vi "Recieve Idot Result.vi"(8 "error in (no error)":errorcluster, 10 "Idot data":waveform(dbl)[](array[waveform]), 11 "Cap Bank Server in":refnum<class "Cap Bank Server.lvclass">) -> (0 "error out":errorcluster, 3 "Cap Bank Server out":refnum<class "Cap Bank Server.lvclass">)   [LabVIEW 2015, in "Cap Bank Server.lvclass"]
uses:
  Cap Bank Server.lvclass
  File/Controls/File formats.ctl
  <vilib>/ActorFramework/Actor/Actor.lvclass/Actor.ctl
  <vilib>/ActorFramework/Message Enqueuer/Message Enqueuer.lvclass/Message Enqueuer.ctl
  Cap Bank Server.lvclass/Cap Bank Server.ctl
  Cap Bank Server Messages/Match idot to shot Msg/Match idot to shot Msg.lvclass/Match idot to shot Msg.ctl
  Mag Lab Measure Controller Messages/Log Status Update Msg/Log Status Update Msg.lvclass/Log Status Update Msg.ctl
  <vilib>/ActorFramework/Message Enqueuer/Init from Existing Queue.vi
  <vilib>/ActorFramework/Message Enqueuer/Enqueue.vi
  <vilib>/ActorFramework/Message Priority Queue/Priority Enqueue.vi
  <vilib>/ActorFramework/Time-Delayed Send Message/Time-Delayed Send Message.vi
  <vilib>/ActorFramework/Message Enqueuer/Message Enqueuer.lvclass
  Mag Lab Measure Controller Messages/Log Status Update Msg/Log Status Update Msg.lvclass
  Cap Bank Server Messages/Match idot to shot Msg/Match idot to shot Msg.lvclass
  <vilib>/ActorFramework/Actor/Actor.lvclass
  Mag Lab Error Handler/Mag Lab Error Handler.lvclass
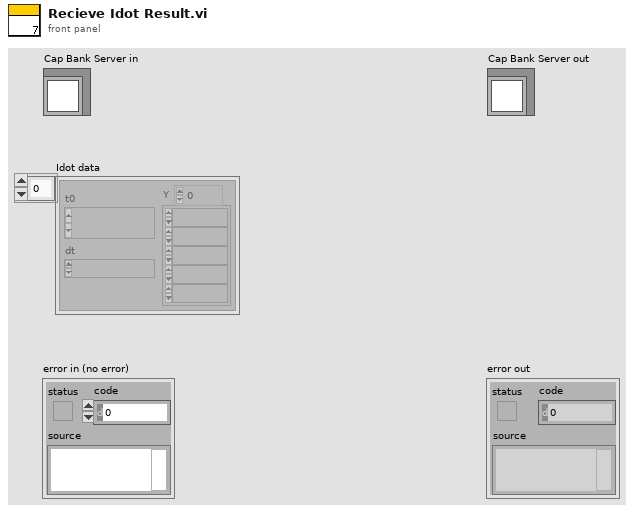
[diagram p1: front panel]
types:
  T1 = enum16{"open", "open or create", "create or replace", "create", "open (read-only)"}
  T2 = typedef "File formats.ctl" = enum16{"TDMS", "ASCII", "BINARY"}
  T3 = cluster{"file path out":path, "Current time":timestamp, i32, dbl}
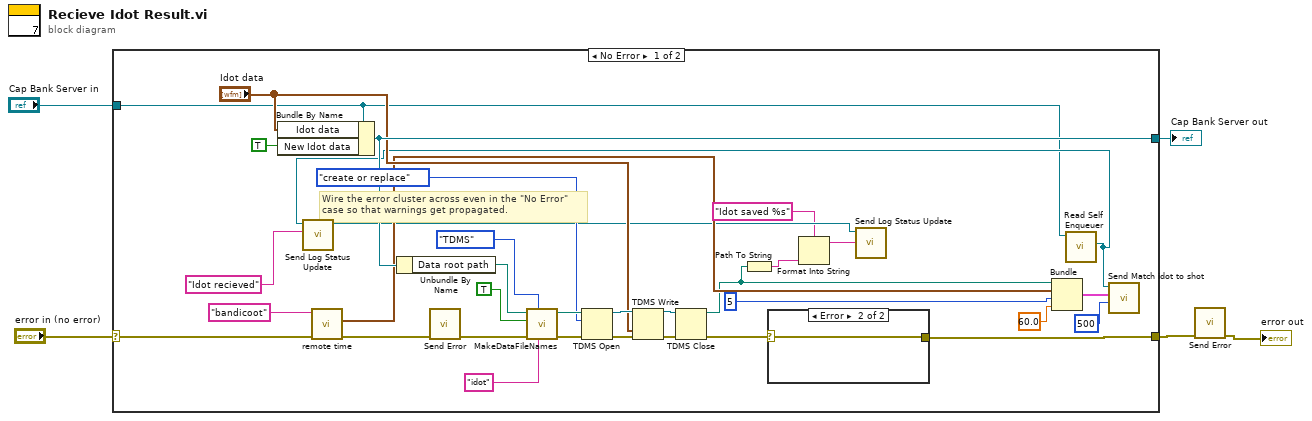
[diagram p0: block diagram]
diagram:
  n1 = case shown="No Error" "error in (no error)" {
    selector: "error in (no error)" -> [w24 w42]
    tunnel: [w15 w42] -> w2
    tunnel: [w37 w41] -> w3
    tunnel: "Cap Bank Server in" -> [w11 w41]
    frame No Error {
      # "Wire the error cluster across even in the \"No Error\"\ncase so that warnings get propagated."
      n2 = Bundle By Name(cluster=w11, "Idot data"="Idot data", "New Idot data"=TRUE) -> (w37:refnum<class "Cap Bank Server.lvclass">)
      n3 = call "remote time.vi"("Error In"=w24, "server"="bandicoot" ("command line")) -> ("Error Out"=w19:errorcluster, "Current time"=w14:timestamp)  [unwired: 6 in, 2 out]
      n4 = Unbundle By Name(w37) -> ("Data root path"=w29:path)
      n5 = call "Send Error.vi"("error in (no error)"=w19) -> ("error out"=w18:errorcluster)  [unwired: 9 in, 1 out]
      n6 = call "MakeDataFileNames.vi"("File Prefix"="idot", "File format"=File_formats."TDMS", "Error In"=w18, "Generate Index"=TRUE, "Root Data Folder"=w29) -> ("Error Out"=w30:errorcluster, "Data File  Path"=w34:path)  [unwired: 3 in, 2 out]
      n7 = TDMS Open(8:w30, 10:T1."create or replace" ("operation (0:open)"), 11:w34) -> (0:w31:errorcluster, 3:w32:refnum<k34>)  [unwired: 4 in]
      n8 = TDMS Write(0:w32, 9:"Idot data", 11:w31) -> (4:w26:refnum<k34>, 15:w27:errorcluster)  [unwired: 3 in, 2 out]
      n9 = TDMS Close(8:w27, 11:w26) -> (0:w16:errorcluster, 3:w9:path)
      n10 = Path To String(path=w9) -> (string=w8:string)
      n11 = case shown="Error" w16 {
        selector: w16 -> [w39 w40]
        tunnel: [w39 w40] -> w15
        frame No Error {
        }
        frame Error {
        }
      }
      n12 = Format Into String(format string="Idot saved %s", w8) -> (resulting string=w6:string)  [unwired: 2 in, 1 out]
      n13 = Bundle("file path out"=w9, "Current time"=w14, 5, 60.0) -> (w20:T3)  [unwired: 1 in]
      n14 = call <vilib>:"Read Self Enqueuer.vi"("Actor"=w11) -> ("Self Enqueuer"=w12:refnum<class "Message Enqueuer.lvclass">)  [unwired: 10 in]
      n15 = call "Send Log Status Update.vi"("Status"="Idot recieved", "Message Enqueuer"=w12) -> ("Message Enqueuer out"=w10:refnum<class "Message Enqueuer.lvclass">)  [unwired: 8 in, 1 out]
      n16 = call "Send Log Status Update.vi"("Status"=w6, "Message Enqueuer"=w10) -> ()  [unwired: 8 in, 2 out]
      n17 = call "Send Match idot to shot.vi"("Delay message, ms"=500, "Idot match record"=w20, "Message Enqueuer"=w12) -> ()  [unwired: 7 in, 2 out]
    }
    frame Error {
    }
  }
  "Cap Bank Server out" <- w3
  n18 = call "Send Error.vi"("error in (no error)"=w2) -> ("error out"=→"error out":errorcluster)  [unwired: 9 in, 1 out]
